vi "TDMS_DEVEL.vi"() -> ()   [LabVIEW 2019]
panel:
  out "Array":i32[](array[numeric])
  in  "Generate Data":bool
  in  "stop":bool
  in  "Write TDMS File":bool
  in  "Test Subject Name":string
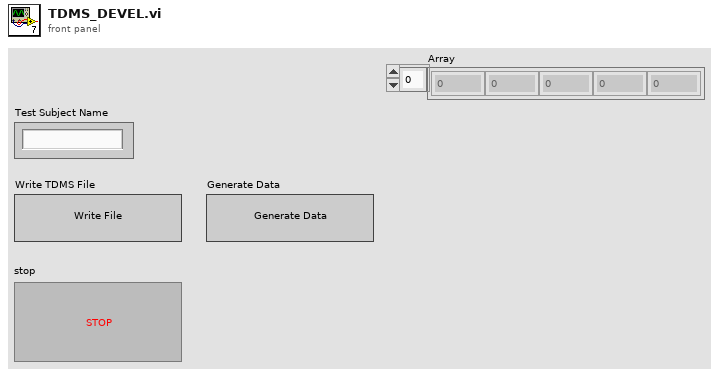
[diagram p1: front panel]
types:
  T1 = enum16{"open", "open or create", "create or replace", "create", "open (read-only)"}
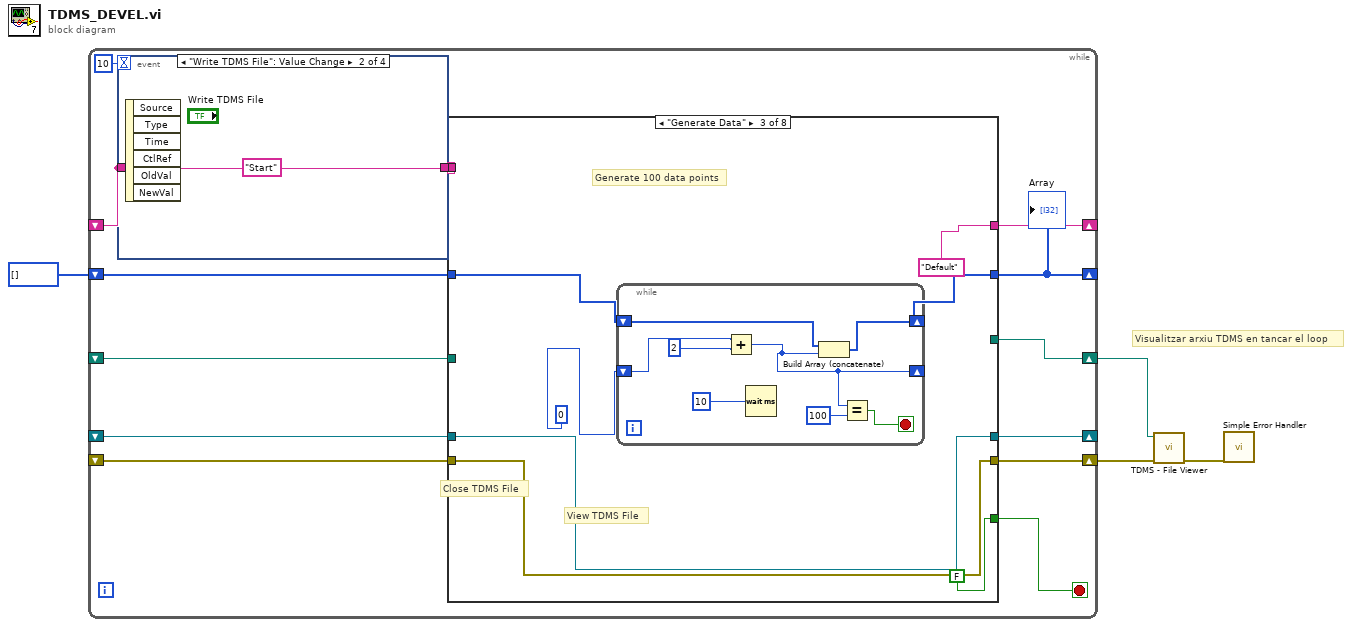
[diagram p0: block diagram]
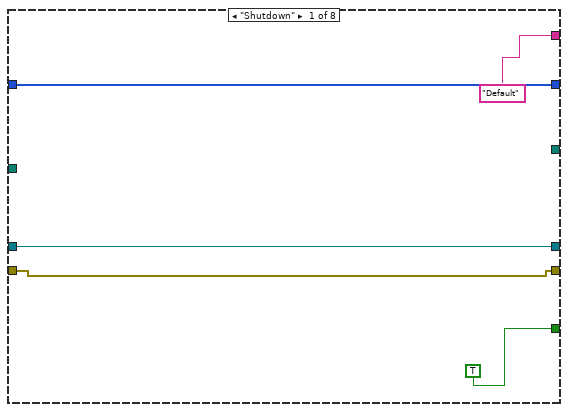
[diagram p2: hidden frame]
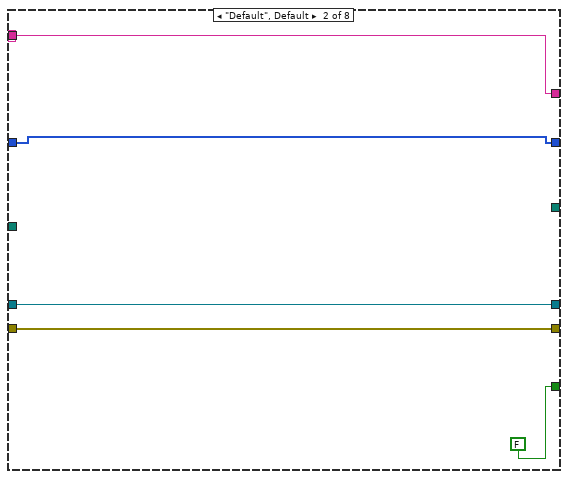
[diagram p3: hidden frame]
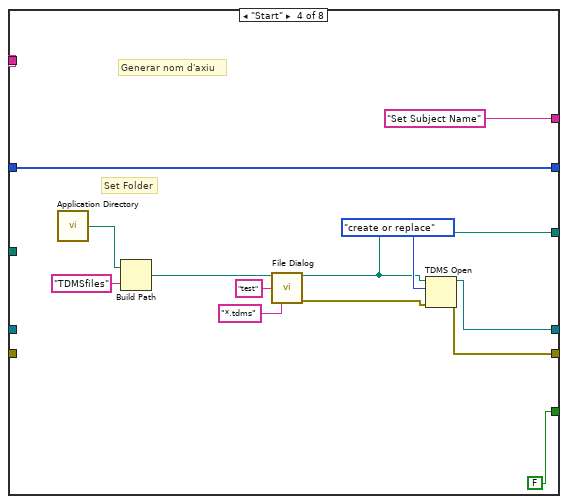
[diagram p4: hidden frame]
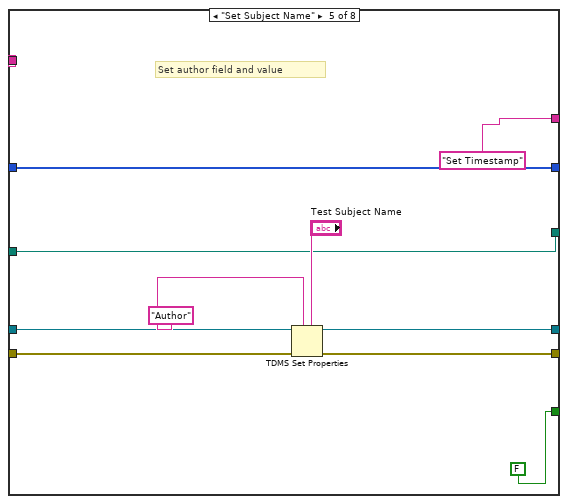
[diagram p5: hidden frame]
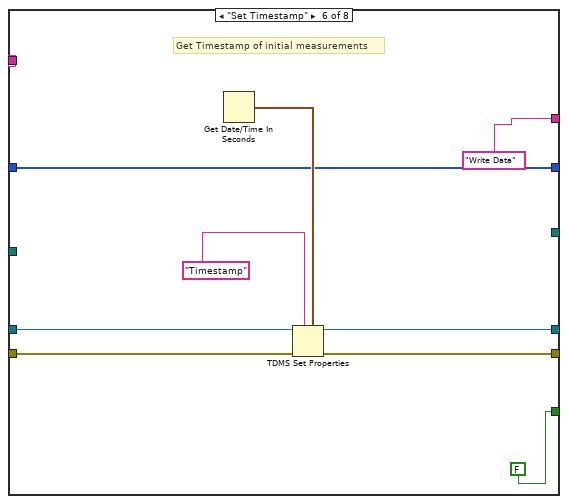
[diagram p6: hidden frame]
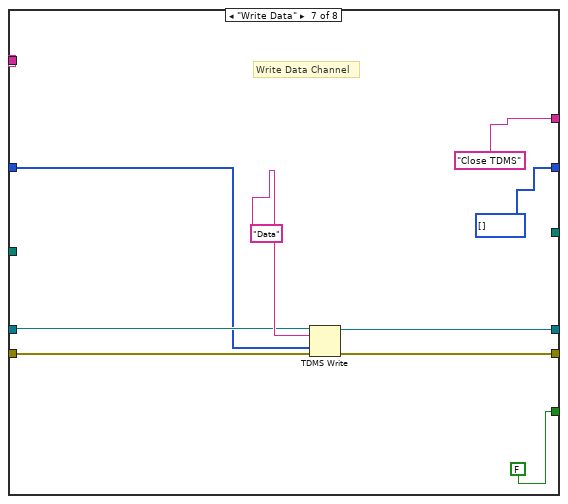
[diagram p7: hidden frame]
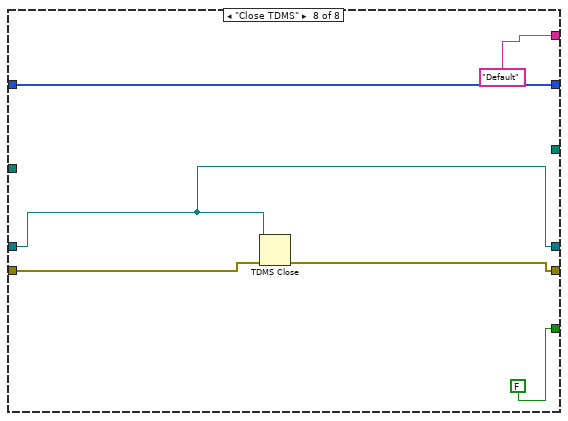
[diagram p8: hidden frame]
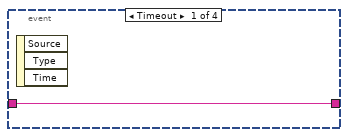
[diagram p9: hidden frame]
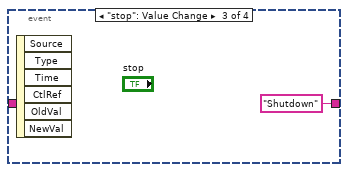
[diagram p10: hidden frame]
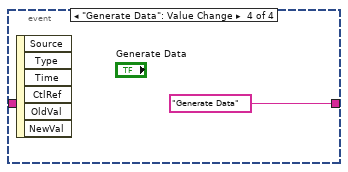
[diagram p11: hidden frame]
diagram:
  # "Visualitzar arxiu TDMS en tancar el loop"
  # "View TDMS File"
  # "Close TDMS File"
  n1 = while {
    shift-right: [w17] -> _
    shift-left: _ -> [w12]
    shift-right: [w16] -> w3
    shift-left: _ -> [w11]
    shift-right: [w15] -> _
    shift-left: _ -> [w13]
    shift-right: [w10] -> _
    shift-left: i32[] [] -> [w9]
    shift-right: [w6] -> w1
    shift-left: _ -> [w5]
    stop <- w8 stop-if-true
    n2 = event shown="[1] \"Write TDMS File\": Value Change" {
      selector: _ -> [_ _ _ _]
      dyn-events: _ -> [_ _ _ _]
      timeout: 10 -> [_ _ _ _]
      tunnel: [w90 "Start" "Shutdown" "Generate Data"] -> w14
      tunnel: w13 -> [w90 _ _ _]
      event Timeout {
        n3 = event-data() -> ()  [unwired: 1 in, 3 out]
      }
      event "Write TDMS File": Value Change {
        n4 = event-data() -> ()  [unwired: 1 in, 6 out]
      }
      event "stop": Value Change {
        n5 = event-data() -> ()  [unwired: 1 in, 6 out]
      }
      event "Generate Data": Value Change {
        n6 = event-data() -> ()  [unwired: 1 in, 6 out]
      }
    }
    n7 = case shown="\"Generate Data\"" w13 {
      tunnel: [w20 w25 w30 w45 w61 w71 w81 w89] -> w16
      tunnel: [w21 w26 w31 w46 w62 w70 w80 w87] -> w17
      tunnel: ["Default" w27 "Default" "Set Subject Name" "Set Timestamp" "Write Data" "Close TDMS" "Default"] -> w15
      tunnel: w14 -> [_ w27 _ _ _ _ _ _]
      tunnel: w12 -> [w21 w26 w31 _ w63 w69 w79 w87]
      tunnel: w11 -> [w20 w25 w30 _ w60 w72 w82 w88]
      tunnel: [w22 w24 w33 w54 w58 w67 i32[] [] w85] -> w10
      tunnel: w9 -> [w22 w24 w29 w54 w58 w67 w77 w85]
      tunnel: [TRUE FALSE FALSE FALSE FALSE FALSE FALSE FALSE] -> w8
      tunnel: [_ _ _ w43 w56 _ _ _] -> w6
      tunnel: w5 -> [_ _ _ _ w56 _ _ _]
      frame "Shutdown" {
      }
      frame "Default", Default {
      }
      frame "Generate Data" {
        # "Generate 100 data points"
        n8 = while {
          shift-right: [w41] -> w33
          shift-left: w29 -> [w40]
          shift-right: [w35] -> _
          shift-left: 0 ("x") -> [w37]
          stop <- w39 stop-if-true
          n9 = Add(x=w37, y=2) -> (x+y=w35:i32)
          n10 = Wait (ms)(milliseconds to wait=u32 10) -> ()  [unwired: 1 out]
          n11 = Build Array (concatenate)(w40, w35) -> (w41:i32[])
          n12 = Equal?(x=w35, y=100) -> (x = y?=w39:bool)
        }
      }
      frame "Start" {
        # "Set Folder"
        # "Generar nom d'axiu"
        n13 = call <vilib>:"Application Directory.vi"() -> ("Application Directory"=w52:path)
        n14 = Build Path(base path=w52, name or relative path="TDMSfiles") -> (appended path=w50:path)
        n15 = call "File Dialog"("start path"=w50, "default name"="test", "pattern (all files)"="*.tdms") -> ("selected path"=w43:path, "error out"=w47:errorcluster)  [unwired: 9 in, 2 out]
        n16 = TDMS Open(8:w47, 10:T1."create or replace" ("operation (0:open)"), 11:w43) -> (0:w45:errorcluster, 3:w46:refnum<k34>)  [unwired: 4 in]
      }
      frame "Set Subject Name" {
        # "Set author field and value"
        n17 = TDMS Set Properties(5:"Test Subject Name", 7:"Author" ("group name"), 8:w60, 11:w63) -> (0:w61:errorcluster, 3:w62:refnum<k34>)  [unwired: 2 in, 2 out]
      }
      frame "Set Timestamp" {
        # "Get Timestamp of initial measurements"
        n18 = Get Date/Time In Seconds() -> (seconds since 1Jan1904=w73:timestamp)
        n19 = TDMS Set Properties(5:w73, 7:"Timestamp" ("group name"), 8:w72, 11:w69) -> (0:w71:errorcluster, 3:w70:refnum<k34>)  [unwired: 2 in, 2 out]
      }
      frame "Write Data" {
        # "Write Data Channel"
        n20 = TDMS Write(0:w79, 5:"Data" ("group name in (Untitled)"), 9:w77, 11:w82) -> (4:w80:refnum<k34>, 15:w81:errorcluster)  [unwired: 2 in, 2 out]
      }
      frame "Close TDMS" {
        n21 = TDMS Close(8:w88, 11:w87) -> (0:w89:errorcluster)  [unwired: 1 out]
      }
    }
    "Array" <- w10
  }
  n22 = call <vilib>:"TDMS - File Viewer.vi"("error in (no error)"=w3, "file path"=w1) -> ("error out"=w2:errorcluster)  [unwired: 4 in, 1 out]
  n23 = call <vilib>:"Simple Error Handler.vi"("error in (no error)"=w2) -> ()  [unwired: 4 in, 5 out]
